vi "SaturationMagnetizationPython.vi"(3 "B":dbl[](array[numeric]), 5 "H":dbl[](array[numeric]), 6 "all gradients":dbl[](array[numeric])) -> (0 "Saturation Field":dbl)   [LabVIEW 2019]
panel:
  out "min index(es)":i32
  out "min value":dbl
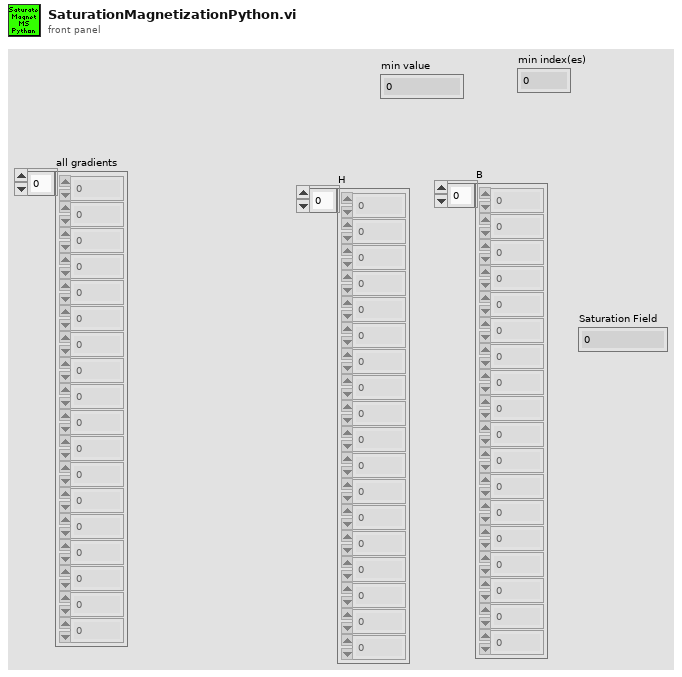
[diagram p1: front panel]
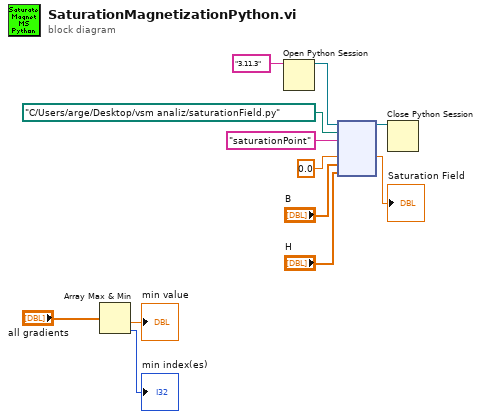
[diagram p0: block diagram]
diagram:
  n1 = Array Max & Min(array="all gradients") -> (min value=→"min value":dbl, min index (indices)=→"min index(es)":i32)  [unwired: 2 out]
  n2 = Open Python Session(python version="3.11.3" ("Python version")) -> (session out=w9:refnum<k35>)  [unwired: 2 in, 1 out]
  n3 = node(w9, path "C:/Users/arge/Desktop/vsm analiz/saturationField.py" ("module path"), "saturationPoint" ("function name"), 0.0, "B", "H") -> (w1:refnum<k35>, →"Saturation Field":dbl)  [unwired: 3 in, 3 out]
  n4 = Close Python Session(session in=w1) -> ()  [unwired: 1 in, 1 out]
